vi "Add VI to Project.vi"(8 "error in":errorcluster, 10 "Project Name":string, 11 "Reference of newly created VI or CTL":refnum<vi>) -> (0 "error out":errorcluster)   [LabVIEW 2022 SP3]
doc: "This VI adds the newly created VI or CTL to a project (lvproj).\n\nThis VI assumes that the newly created VI has already been saved to disk (already exists on disk)."
panel:
  # "Development\ncontrols/indicators useful for development and testing, but which are not outputs of the VI"
  # "Input\nInputs to the VI"
  # "Output\nOutputs of the VI"
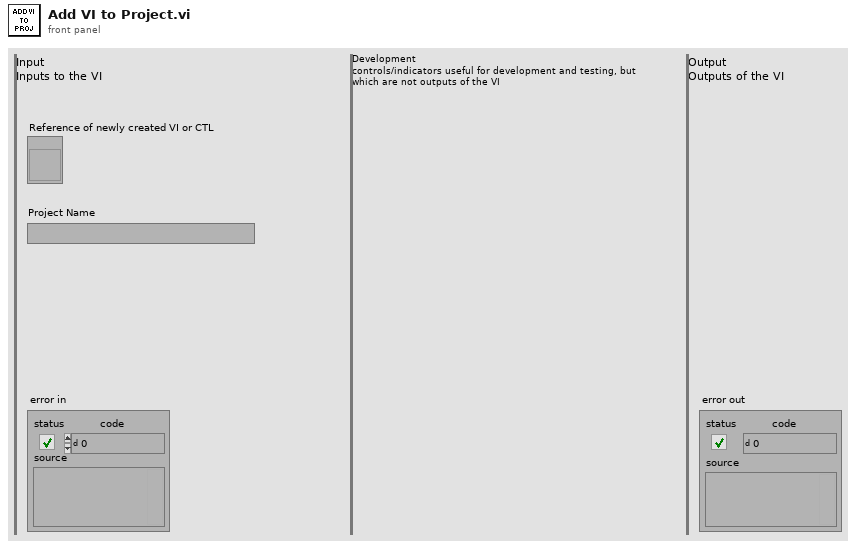
[diagram p1: front panel]
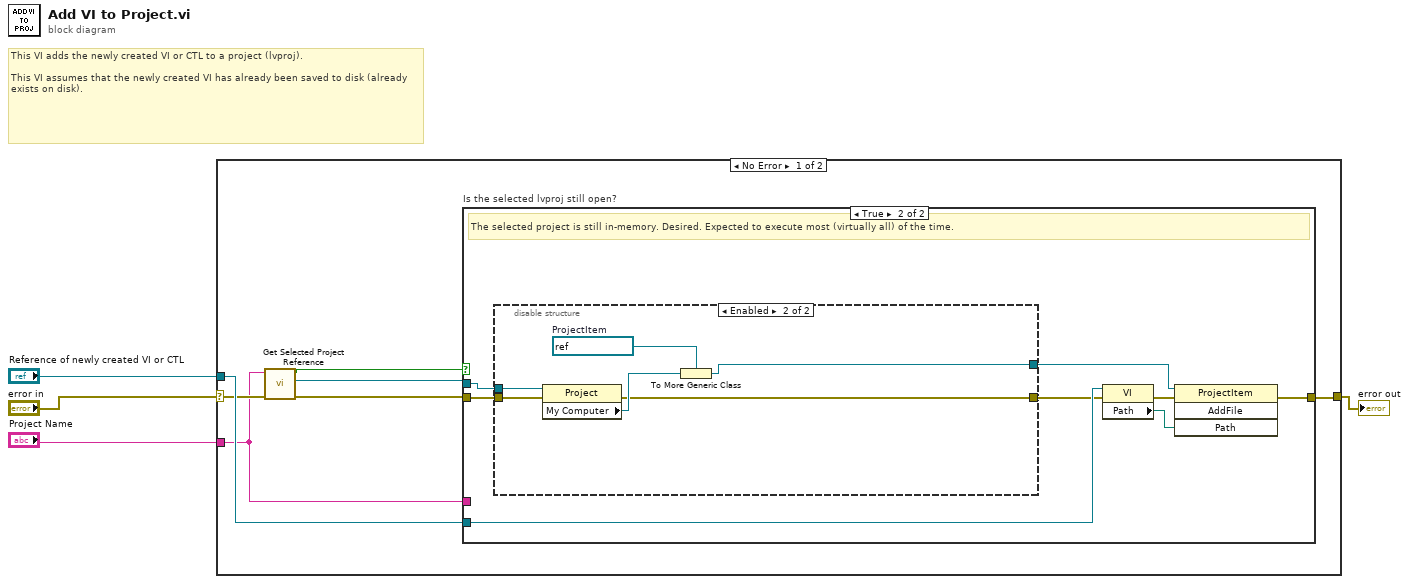
[diagram p0: block diagram]
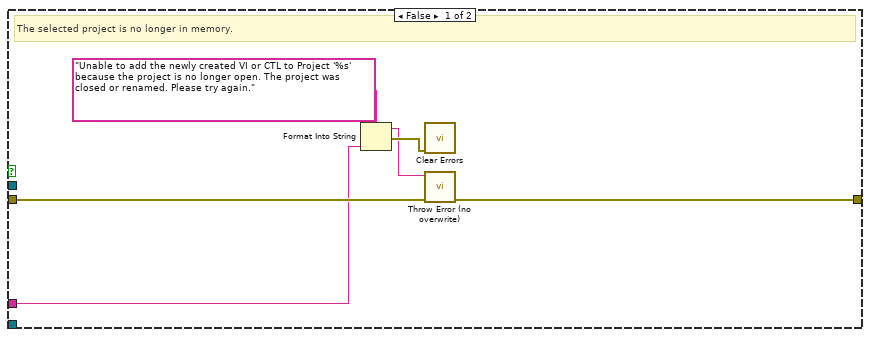
[diagram p2: hidden frame]
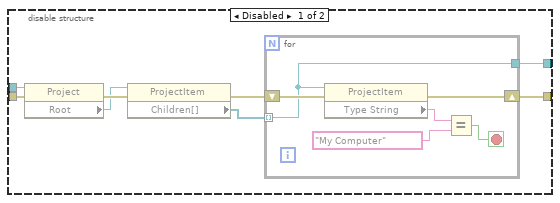
[diagram p3: hidden frame]
diagram:
  # "This VI adds the newly created VI or CTL to a project (lvproj).\n\nThis VI assumes that the newly created VI has already been saved to disk (already exists on disk)."
  n1 = case shown="No Error" "error in" {
    selector: "error in" -> [w9 w46]
    tunnel: [w11 w46] -> w3
    tunnel: "Reference of newly created VI or CTL" -> [w10 _]
    tunnel: "Project Name" -> [w8 _]
    frame No Error {
      n2 = call "Get Selected Project Reference.vi"("error in"=w9, "Selected Project Name"=w8) -> ("error out"=w7:errorcluster, "Project Refnum"=w6:refnum<vi>, "Was Project Found?"=w5:bool)  [unwired: 7 in]
      n3 = case "Is the selected lvproj still open?" shown="True" w5 {
        tunnel: [w16 w23] -> w11
        tunnel: w7 -> [w17 w25]
        tunnel: w6 -> [_ w24]
        tunnel: w10 -> [_ w22]
        tunnel: w8 -> [w13 _]
        frame False {
          # "The selected project is no longer in memory."
          n4 = Format Into String(format string="Unable to add the newly created VI or CTL to Project '%s' because the project is no longer open. The project was closed or renamed. Please try again." ("message"), w13) -> (resulting string=w12:string, error out=w14:errorcluster)  [unwired: 2 in]
          n5 = call <vilib>:"Clear Errors.vi"("error in (no error)"=w14) -> ()  [unwired: 5 in, 2 out]
          n6 = call "Throw Error (no overwrite).vi"("error in"=w17, "Error Message"=w12) -> ("error out"=w16:errorcluster)  [unwired: 9 in]
        }
        frame True {
          # "The selected project is still in-memory. Desired. Expected to execute most (virtually all) of the time."
          n7 = disable-structure shown="Enabled" {
            disable-tunnel: w25 -> [w33 w45]
            disable-tunnel: w24 -> [w31 w44]
            disable-tunnel: [w27 w41] -> w20
            disable-tunnel: [w26 w40] -> w19
            frame Disabled {
              n8 = property class="Project"(reference=w31, error in=w33) -> (error out=w32:errorcluster, "Root"=w30:refnum<vi>)  [unwired: 1 out]
              n9 = property class="ProjectItem"(reference=w30, error in=w32) -> (error out=w29:errorcluster, "Children[]"=w28:refnum<vi>[])  [unwired: 1 out]
              n10 = for {
                shift-right: [w38] -> w26
                shift-left: w29 -> [w39]
                tunnel: w28 -> [w34] mode=indexing
                tunnel: [w34] -> w27
                stop <- w35 stop-if-true
                n11 = property class="ProjectItem"(reference=w34, error in=w39) -> (error out=w38:errorcluster, "Type String"=w37:string)  [unwired: 1 out]
                n12 = Equal?(x=w37, y="My Computer") -> (x = y?=w35:bool)
              }
            }
            frame Enabled {
              w42 = refnum<vi> refnum  # ProjectItem
              n13 = property class="Project"(reference=w44, error in=w45) -> (error out=w40:errorcluster, "My Computer"=w43:refnum<vi>)  [unwired: 1 out]
              n14 = To More Generic Class(target class=w42, reference=w43) -> (generic class reference=w41:refnum<vi>)
            }
          }
          n15 = property class="VI"(reference=w22, error in=w19) -> (error out=w18:errorcluster, "Path"=w21:path)  [unwired: 1 out]
          n16 = invoke class="ProjectItem" method="AddFile"(reference=w20, error in=w18, "Path"=w21) -> (error out=w23:errorcluster)  [unwired: 1 in, 3 out]
        }
      }
    }
    frame Error {
    }
  }
  "error out" <- w3
